vi "Load.vi"(8 "error in":errorcluster) -> (0 "error out":errorcluster, 3 "Data out":T1)   [LabVIEW 2015, in "Main INI.lvlib"]
uses:
  Main INI.lvlib
  Core Data.ctl
  Action.ctl
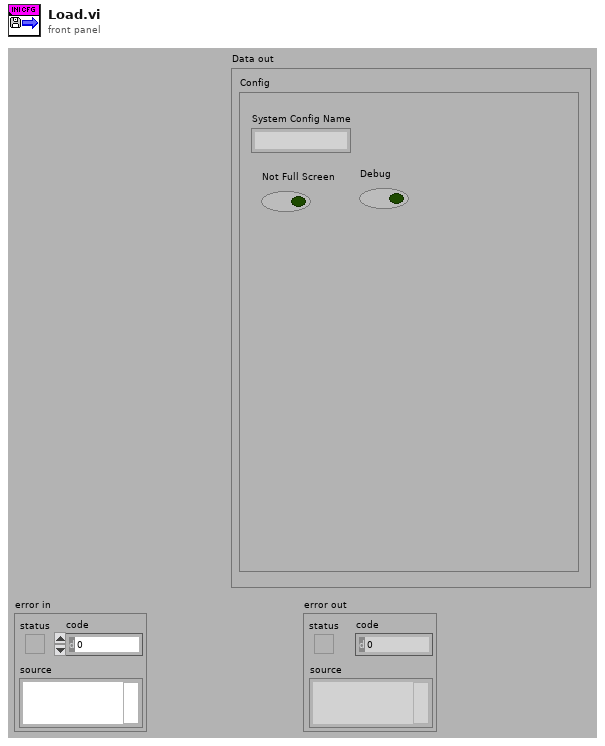
[diagram p1: front panel]
types:
  T1 = typedef "Main INI.lvlib/Core Data.ctl" = cluster{"Config":cluster{"System Config Name":string, "Not Full Screen":bool, "Debug":bool}}
  T2 = typedef "Main INI.lvlib/Action.ctl" = enum16{"Initialise", "Save", "Load", "get All", "set System Config"}
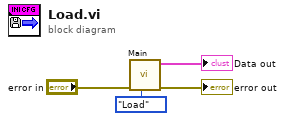
[diagram p0: block diagram]
diagram:
  n1 = call "Main.vi"("Action (get)"=Action."Load", "error in"="error in") -> ("error out"=→"error out":errorcluster, "Data out"=→"Data out":T1)  [unwired: 8 in]
